vi "Test.vi"(6 "error in":errorcluster, 7 "array":bool[][](array[boolean]), 8 "Количество датчиков":i32, 9 "Номер иттерации":i32, 11 "task/channels in":refnum<k21>) -> (0 "Индекс переключаемого канала":i32, 1 "error out":errorcluster, 3 "task out":refnum<k21>, 4 "Что следует из алгоритма":bool[](array[boolean]))   [LabVIEW 2018]
doc: "Подприбор обеспечивает переключение реле, согласно переданному boolean массиву"
uses:
  <vilib>/DAQmx/write.llb/DAQmx Write (Digital 1D Bool NChan 1Samp 1Line).vi
  <vilib>/DAQmx/miscellaneous.llb/DAQmx Fill In Error Info.vi
panel:
  # "Период перключения"
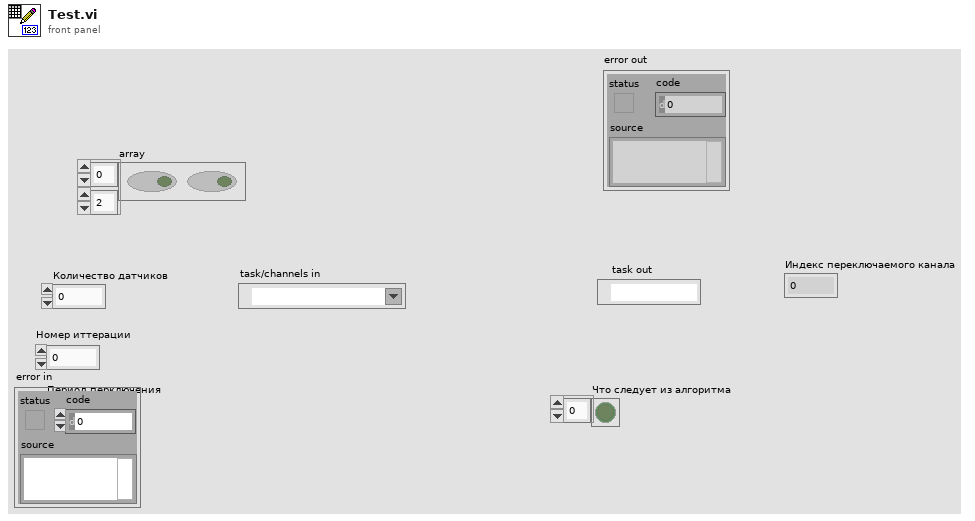
[diagram p1: front panel]
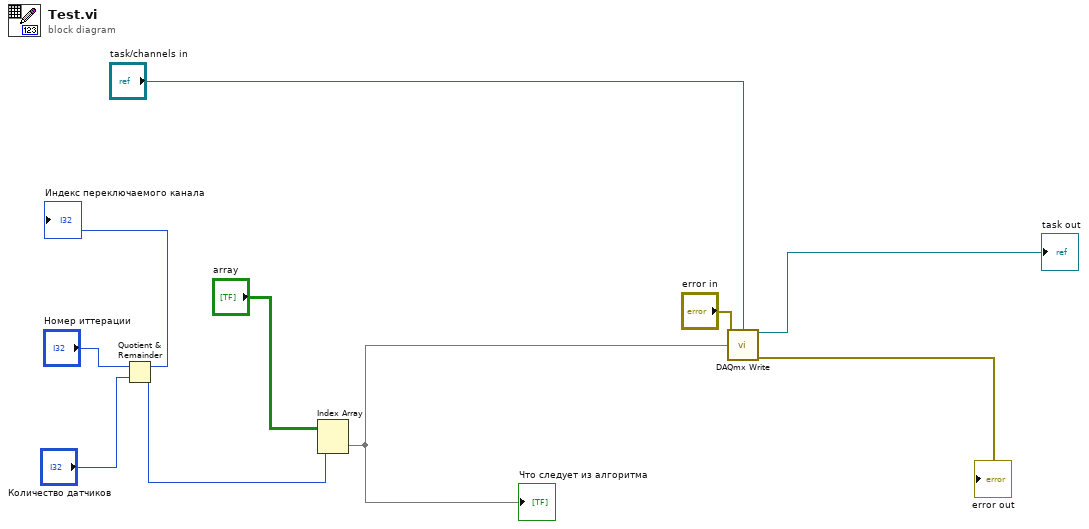
[diagram p0: block diagram]
diagram:
  n1 = Quotient & Remainder(x="Номер иттерации", y="Количество датчиков") -> (x-y*floor(x/y)=w3:i32)  [unwired: 1 out]
  "Индекс переключаемого канала" <- w3
  n2 = Index Array(array="array", index (col)=w3) -> (element=w4:bool[])  [unwired: 1 in]
  "Что следует из алгоритма" <- w4
  n3 = call-poly <vilib>:"DAQmx Write.vi"("task/channels in"="task/channels in", "data"=w4, "error in"="error in") -> ("task out"=→"task out":refnum<k21>, "error out"=→"error out":errorcluster)  [unwired: 10 in, 1 out]
